vi "Get Parameter Definition.vi"(8 "error in":errorcluster, 11 "parameter":T2 format="%.0x") -> (0 "error out":errorcluster, 2 "parameter definition":T1, 3 "parameter out":T2 format="%.0x")   [LabVIEW 2020, in "AIM MIL-STD-1553 Scripting.lvlib"]
doc: "Returns the <b>parameter definition</b> for the input <b>parameter</b>."
uses:
  AIM MIL-STD-1553 Scripting.lvlib
  <vilib>/NI VeriStand/Custom Device API/Custom Device Item Ref.ctl
  Shared/Parameter Definition.ctl
  Constants.vi
  <vilib>/NI VeriStand/Custom Device API/Get Item Property (I32).vi
  <vilib>/NI VeriStand/Custom Device API/Get Item Property (U16).vi
  <vilib>/NI VeriStand/Custom Device API/Get Item Property (Boolean).vi
  <vilib>/NI VeriStand/Custom Device API/Get Item Property (Double).vi
  <vilib>/NI VeriStand/Custom Device API/Custom Device API.lvlib
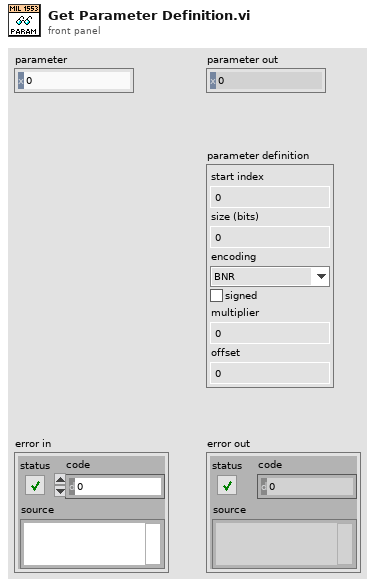
[diagram p1: front panel]
types:
  T1 = typedef "Parameter Definition.ctl" = cluster{"start index":i32, "size (bits)":i32, "encoding":enum16{"BNR", "BCD", "Discrete"}, "signed":bool, "multiplier":dbl, "offset":dbl}
  T2 = typedef "Custom Device API.lvlib/Custom Device Item Ref.ctl" = u64
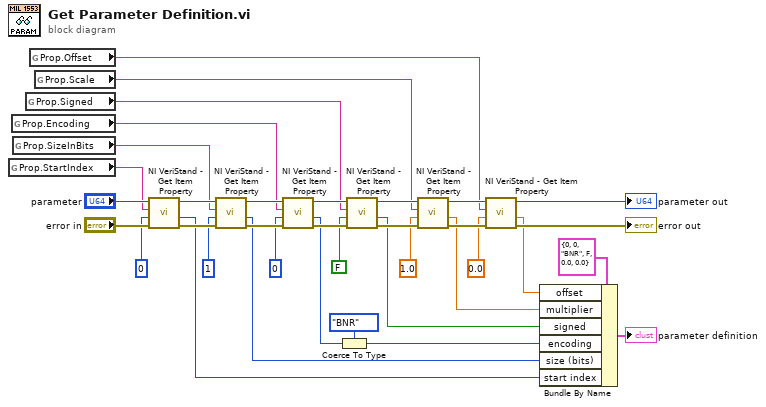
[diagram p0: block diagram]
diagram:
  n1 = global read "Constants.vi" "Prop.StartIndex"() -> (w15:string)
  n2 = global read "Constants.vi" "Prop.Encoding"() -> (w17:string)
  n3 = global read "Constants.vi" "Prop.SizeInBits"() -> (w16:string)
  n4 = global read "Constants.vi" "Prop.Signed"() -> (w18:string)
  n5 = global read "Constants.vi" "Prop.Offset"() -> (w20:string)
  n6 = global read "Constants.vi" "Prop.Scale"() -> (w19:string)
  n7 = call-poly <vilib>:"NI VeriStand - Get Item Property.vi"("error in (no error)"="error in", "Default Value"=0, "Property Name"=w15, "Item Ref in"="parameter") -> ("error out"=w33:errorcluster, "Value"=w3:i32, "Item Ref out"=w34:T2)  [unwired: 4 in, 1 out]
  n8 = call-poly <vilib>:"NI VeriStand - Get Item Property.vi"("error in (no error)"=w33, "Default Value"=1, "Property Name"=w16, "Item Ref in"=w34) -> ("error out"=w31:errorcluster, "Value"=w5:i32, "Item Ref out"=w32:T2)  [unwired: 4 in, 1 out]
  n9 = call-poly <vilib>:"NI VeriStand - Get Item Property.vi"("error in (no error)"=w31, "Default Value"=u16 0, "Property Name"=w17, "Item Ref in"=w32) -> ("error out"=w29:errorcluster, "Value"=w7:u16, "Item Ref out"=w30:T2)  [unwired: 4 in, 1 out]
  n10 = Coerce To Type(0:w7, 1:enum16{"BNR", "BCD", "Discrete"}."BNR" ("parameter definition.encoding")) -> (2:w35:enum16{"BNR", "BCD", "Discrete"})
  n11 = call-poly <vilib>:"NI VeriStand - Get Item Property.vi"("error in (no error)"=w29, "Default Value"=FALSE ("required (F)"), "Property Name"=w18, "Item Ref in"=w30) -> ("error out"=w27:errorcluster, "Value"=w9:bool, "Item Ref out"=w28:T2)  [unwired: 4 in, 1 out]
  n12 = call-poly <vilib>:"NI VeriStand - Get Item Property.vi"("error in (no error)"=w27, "Default Value"=1.0, "Property Name"=w19, "Item Ref in"=w28) -> ("error out"=w25:errorcluster, "Value"=w10:dbl, "Item Ref out"=w26:T2)  [unwired: 4 in, 1 out]
  n13 = call-poly <vilib>:"NI VeriStand - Get Item Property.vi"("error in (no error)"=w25, "Default Value"=0.0, "Property Name"=w20, "Item Ref in"=w26) -> ("error out"=→"error out":errorcluster, "Value"=w12:dbl, "Item Ref out"=→"parameter out":T2)  [unwired: 4 in, 1 out]
  n14 = Bundle By Name(cluster=T1 {"start index"=0, "size (bits)"=0, "encoding"=enum."BNR", "signed"=FALSE, "multiplier"=0.0, "offset"=0.0} ("parameter definition"), "offset"=w12, "multiplier"=w10, "signed"=w9, "encoding"=w35, "size (bits)"=w5, "start index"=w3) -> (→"parameter definition":T1)
